vi "Joystick to Swerve New.vi"(1 "Joystick Y":dbl, 2 "Joystick R":dbl, 3 "Joystick X":dbl) -> (0 "output cluster":T1)   [LabVIEW 2018]
uses:
  Motor Data Unpacked.ctl
panel:
  out "D":dbl
  out "C":dbl
  out "B":dbl
  out "A":dbl
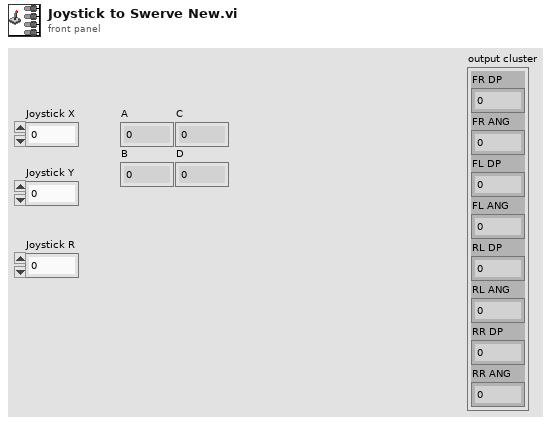
[diagram p1: front panel]
types:
  T1 = typedef "Motor Data Unpacked.ctl" = cluster{"FR DP":dbl, "FR ANG":dbl, "FL DP":dbl, "FL ANG":dbl, "RL DP":dbl, "RL ANG":dbl, "RR DP":dbl, "RR ANG":dbl}
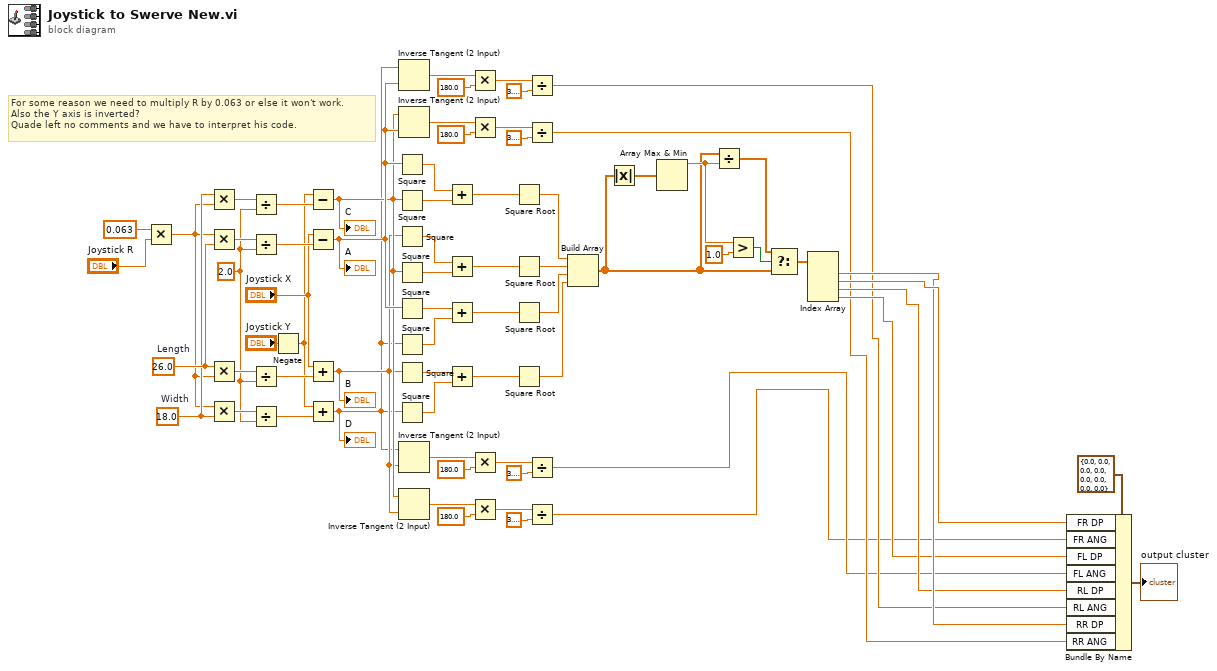
[diagram p0: block diagram]
diagram:
  w32 = 2.0
  w33 = 18.0  # Width
  w68 = 26.0  # Length
  # "For some reason we need to multiply R by 0.063 or else it won't work.\nAlso the Y axis is inverted?\nQuade left no comments and we have to interpret his code."
  n1 = Multiply(x=0.063, y="Joystick R") -> (x*y=w2:dbl)
  n2 = Multiply(x=w33, y=w2) -> (x*y=w65:dbl)
  n3 = Multiply(x=w2, y=w68) -> (x*y=w70:dbl)
  n4 = Multiply(x=w68, y=w2) -> (x*y=w67:dbl)
  n5 = Multiply(x=w2, y=w33) -> (x*y=w63:dbl)
  n6 = Divide(x=w65, y=w32) -> (x/y=w64:dbl)
  n7 = Divide(x=w70, y=w32) -> (x/y=w69:dbl)
  n8 = Divide(x=w67, y=w32) -> (x/y=w66:dbl)
  n9 = Divide(x=w63, y=w32) -> (x/y=w62:dbl)
  n10 = Negate(x="Joystick Y") -> (-x=w4:dbl)
  n11 = Subtract(x=w4, y=w64) -> (x-y=w30:dbl)
  "C" <- w30
  n12 = Subtract(x="Joystick X", y=w69) -> (x-y=w31:dbl)
  "A" <- w31
  n13 = Add(x="Joystick X", y=w66) -> (x+y=w29:dbl)
  "B" <- w29
  n14 = Add(x=w4, y=w62) -> (x+y=w28:dbl)
  "D" <- w28
  n15 = Square(x=w31) -> (x^2=w36:dbl)
  n16 = Square(x=w30) -> (x^2=w35:dbl)
  n17 = Square(x=w29) -> (x^2=w57:dbl)
  n18 = Square(x=w30) -> (x^2=w56:dbl)
  n19 = Square(x=w31) -> (x^2=w43:dbl)
  n20 = Square(x=w28) -> (x^2=w42:dbl)
  n21 = Square(x=w29) -> (x^2=w50:dbl)
  n22 = Square(x=w28) -> (x^2=w49:dbl)
  n23 = Inverse Tangent (2 Input)(1:w31, 2:w28) -> (0:w47:dbl)
  n24 = Inverse Tangent (2 Input)(1:w31, 2:w30) -> (0:w40:dbl)
  n25 = Inverse Tangent (2 Input)(1:w29, 2:w28) -> (0:w54:dbl)
  n26 = Inverse Tangent (2 Input)(1:w29, 2:w30) -> (0:w61:dbl)
  n27 = Add(x=w36, y=w35) -> (x+y=w34:dbl)
  n28 = Add(x=w57, y=w56) -> (x+y=w55:dbl)
  n29 = Add(x=w43, y=w42) -> (x+y=w41:dbl)
  n30 = Add(x=w50, y=w49) -> (x+y=w48:dbl)
  n31 = Multiply(x=w47, y=180.0) -> (x*y=w44:dbl)
  n32 = Multiply(x=w40, y=180.0) -> (x*y=w38:dbl)
  n33 = Multiply(x=w54, y=180.0) -> (x*y=w51:dbl)
  n34 = Multiply(x=w61, y=180.0) -> (x*y=w58:dbl)
  n35 = Square Root(x=w34) -> (sqrt(x)=w27:dbl)
  n36 = Square Root(x=w55) -> (sqrt(x)=w26:dbl)
  n37 = Square Root(x=w41) -> (sqrt(x)=w25:dbl)
  n38 = Square Root(x=w48) -> (sqrt(x)=w24:dbl)
  n39 = Divide(x=w44, y=3.141592653589793) -> (x/y=w11:dbl)
  n40 = Divide(x=w38, y=3.141592653589793) -> (x/y=w10:dbl)
  n41 = Divide(x=w51, y=3.141592653589793) -> (x/y=w9:dbl)
  n42 = Divide(x=w58, y=3.141592653589793) -> (x/y=w8:dbl)
  n43 = Build Array(w27, w26, w25, w24) -> (w18:dbl[])
  n44 = Absolute Value(x=w18) -> (abs(x)=w23:dbl[])
  n45 = Array Max & Min(array=w23) -> (max value=w20:dbl)  [unwired: 3 out]
  n46 = Divide(x=w18, y=w20) -> (x/y=w19:dbl[])
  n47 = Greater?(x=w20, y=1.0) -> (0:w21:bool)
  n48 = Select(t=w19, s=w21, f=w18) -> (s? t:f=w17:dbl[])
  n49 = Index Array(array=w17) -> (element #1=w14:dbl, element #2=w15:dbl, element #3=w13:dbl, element #4=w12:dbl)  [unwired: 4 in]
  n50 = Bundle By Name(cluster=T1 {"FR DP"=0.0, "FR ANG"=0.0, "FL DP"=0.0, "FL ANG"=0.0, "RL DP"=0.0, "RL ANG"=0.0, "RR DP"=0.0, "RR ANG"=0.0}, "FR DP"=w15, "FR ANG"=w8, "FL DP"=w12, "FL ANG"=w9, "RL DP"=w13, "RL ANG"=w11, "RR DP"=w14, "RR ANG"=w10) -> (→"output cluster":T1)
